vi "View Get Duration.vi"(8 "error in (no error)":errorcluster, 11 "Chef View in":refnum<class "Chef View.lvclass">) -> (0 "error out":errorcluster, 2 "Duration":dbl, 3 "Chef View out":refnum<class "Chef View.lvclass">)   [LabVIEW 2024]
uses:
  Chef View.lvclass
  Chef View.lvclass/Chef View.ctl
  C:/Program Files/National Instruments/LabVIEW 2024/vi.lib/ActorFramework/Actor/Actor.lvclass
  G:/Leveling/LabVIEW/Learning/Actor Framework/chef/Chef View/Chef View.lvclass
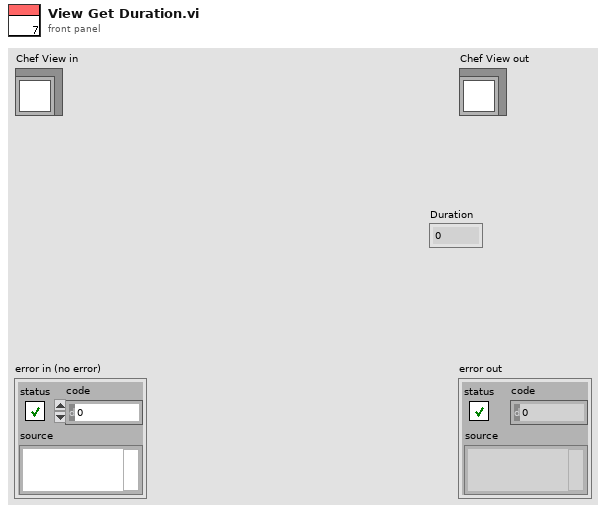
[diagram p1: front panel]
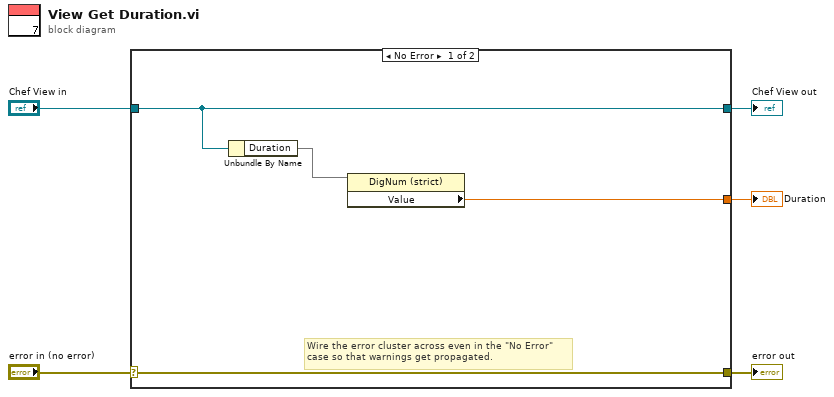
[diagram p0: block diagram]
diagram:
  n1 = case shown="No Error" "error in (no error)" {
    selector: "error in (no error)" -> [w9 w11]
    tunnel: [w9 w11] -> w4
    tunnel: [w8 w10] -> w2
    tunnel: "Chef View in" -> [w8 w10]
    tunnel: [w6 _] -> w1
    frame No Error {
      # "Wire the error cluster across even in the \"No Error\"\ncase so that warnings get propagated."
      n2 = Unbundle By Name(w8) -> ("Duration"=w7)
      n3 = property class="DigNum (strict)"(reference=w7) -> ("Value"=w6:dbl)  [unwired: 1 in, 2 out]
    }
    frame Error {
    }
  }
  "error out" <- w4
  "Chef View out" <- w2
  "Duration" <- w1
